vi "PRIME Telescope Convert HHMMSS string.vi"(10 "RA String":string) -> (1 "Array":dbl[](array[numeric]), 2 "Right Ascension":T1)   [LabVIEW 2021, in "PRIME Telescope.lvclass"]
uses:
  PRIME Telescope.lvclass
  <vilib>/regexp/Match Regular Expression.xnode
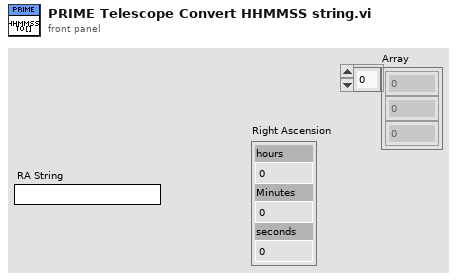
[diagram p1: front panel]
types:
  T1 = cluster{"hours":dbl, "Minutes":dbl, "seconds":dbl}
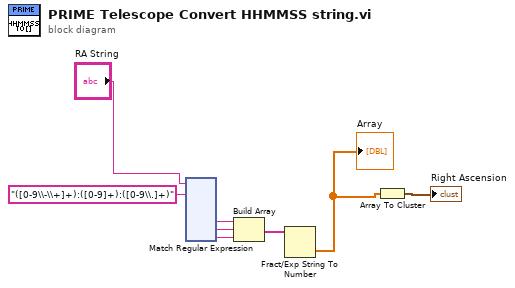
[diagram p0: block diagram]
diagram:
  n1 = xnode "Match Regular Expression"("input string"="RA String", "regular expression"="([0-9\\-\\+]+):([0-9]+):([0-9\\.]+)") -> ("submatch 1"=w7:string, "submatch 2"=w6:string, "submatch 3"=w5:string)  [unwired: 4 in, 5 out]
  n2 = Build Array(w7, w6, w5) -> (w4:string[])
  n3 = Fract/Exp String To Number(string=w4) -> (number=w2:dbl[])  [unwired: 3 in, 1 out]
  "Array" <- w2
  n4 = Array To Cluster(array=w2) -> (cluster=→"Right Ascension":cluster{"[0]":dbl, "[1]":dbl, "[2]":dbl})
